vi "Configure PID Module.vi"(0 "VISA resource name":refnum<visa-resource-name>, 5 "Unit No. (0)":i32 min=0 max=6, 7 "Module No.(0)":i32 min=0 max=9, 9 "Burnout Lower Limit":dbl=-10.0 min=-200.0 max=50.0 format="%.1f", 11 "error in (no error)":errorcluster, 12 "Burnout Upper Limit":dbl=110.0 min=1050.0 max=1200.0 format="%.1f") -> (4 "VISA resource name out":refnum<visa-resource-name>, 8 "Unit No.":i32, 10 "Module No.":i32, 15 "error out":errorcluster)   [LabVIEW 2020, in "Yokogawa GX Series.lvlib"]
doc: "Sets integration time, burnout lower upper limits to specified PID module.\n\nCommand: SModePID"
uses:
  <instrlib>/Yokogawa GX Series/Yokogawa GX Series.lvlib
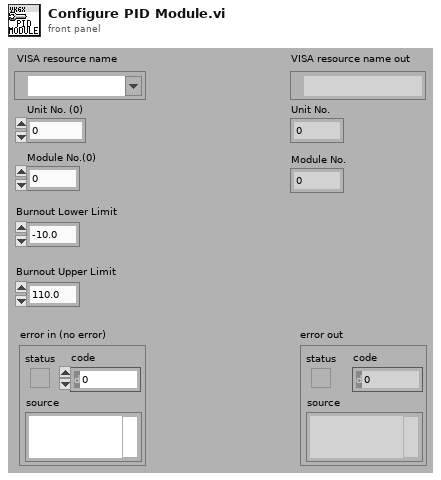
[diagram p1: front panel]
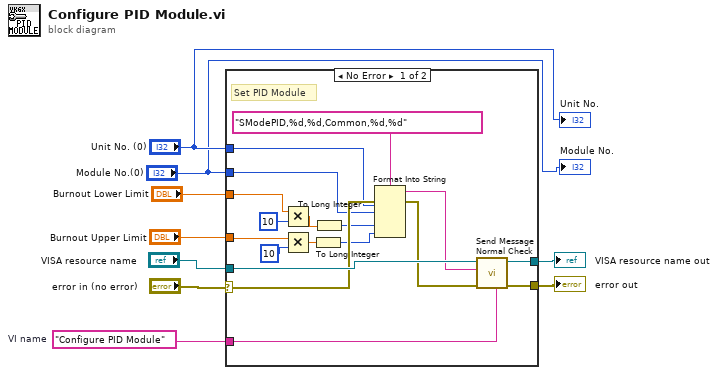
[diagram p0: block diagram]
diagram:
  w5 = "Configure PID Module"  # VI name
  n1 = case shown="No Error" "error in (no error)" {
    selector: "error in (no error)" -> [w22 w28]
    tunnel: [w27 w29] -> w9
    tunnel: [w26 w28] -> w8
    tunnel: "VISA resource name" -> [w25 w29]
    tunnel: w5 -> [w21 _]
    tunnel: "Unit No. (0)" -> [w19 _]
    tunnel: "Module No.(0)" -> [w18 _]
    tunnel: "Burnout Lower Limit" -> [w12 _]
    tunnel: "Burnout Upper Limit" -> [w16 _]
    frame No Error {
      # "Set PID Module"
      n2 = Multiply(x=w12, y=10) -> (x*y=w11:dbl)
      n3 = Multiply(x=w16, y=10) -> (x*y=w15:dbl)
      n4 = To Long Integer(number=w15) -> (32bit integer=w14:i32)
      n5 = To Long Integer(number=w11) -> (32bit integer=w10:i32)
      n6 = Format Into String(format string="SModePID,%d,%d,Common,%d,%d", error in=w22, w19, w18, w10, w14) -> (resulting string=w20:string, error out=w23:errorcluster)  [unwired: 1 in]
      n7 = call <instrlib>:"Send Message Normal Check.vi"("Source (\"\")"=w21, "error in (no error)"=w23, "Send Message (\"\")"=w20, "VISA resource name"=w25) -> ("error out"=w26:errorcluster, "VISA resource name out"=w27:refnum<visa-resource-name>)  [unwired: 2 in, 4 out]
    }
    frame Error {
    }
  }
  "error out" <- w8
  "VISA resource name out" <- w9
  "Unit No." <- "Unit No. (0)"
  "Module No." <- "Module No.(0)"
